vi "CRYSet Import Calibration Data Dialog Front Panel.vi"(11 "Vi Ref":refnum<vi>) -> ()   [LabVIEW 2013]
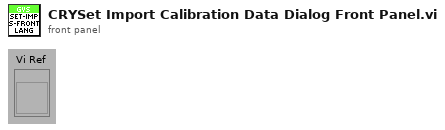
[diagram p1: front panel]
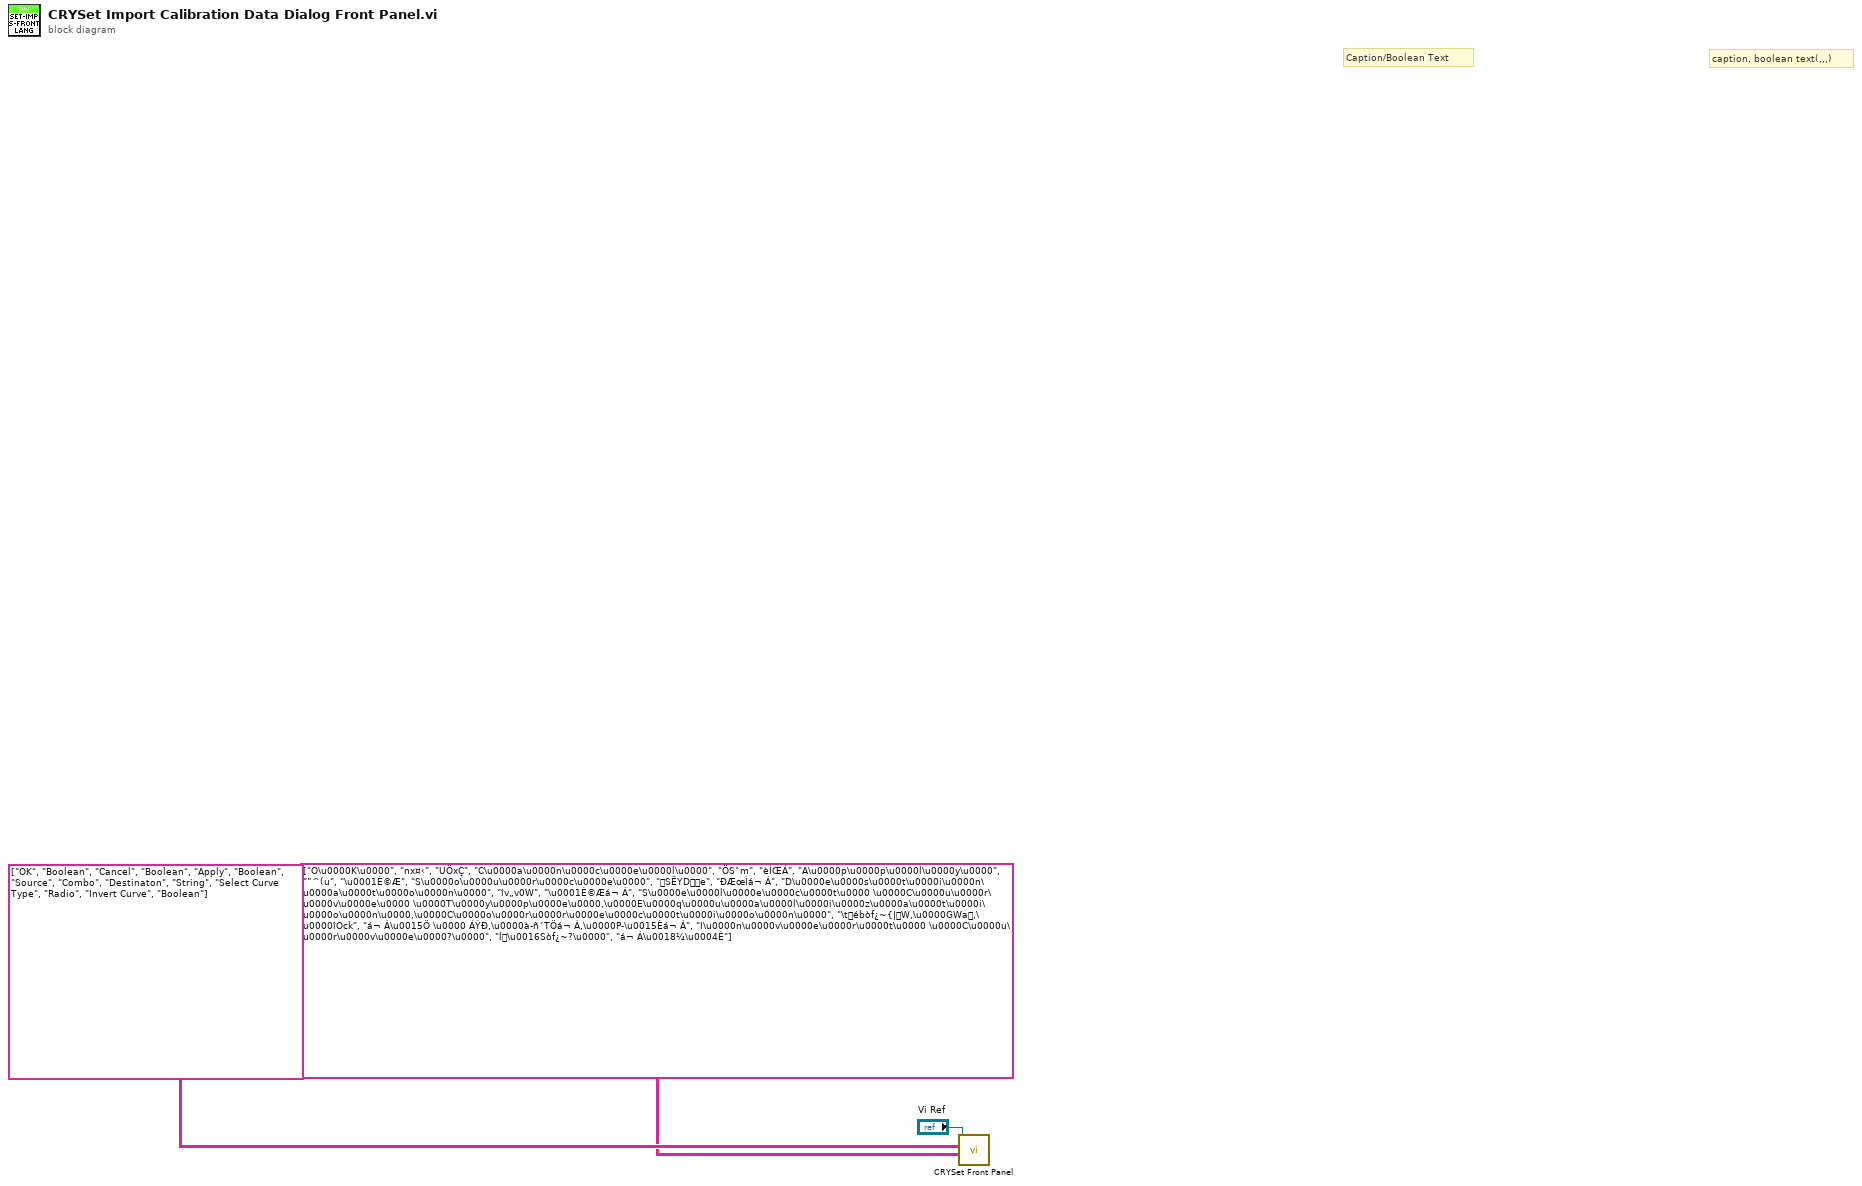
[diagram p0: block diagram]
diagram:
  # "caption, boolean text(,,,)"
  # "Caption/Boolean Text"
  n1 = call "CRYSet Front Panel.vi"("Caption(Boolean Text)"=string[][] [["O\u0000K\u0000", "nx¤‹", "UÖxÇ"], ["C\u0000a\u0000n\u0000c\u0000e\u0000l\u0000", "ÖSˆm", "èÍŒÁ"], ["A\u0000p\u0000p\u0000l\u0000y\u0000", "”^(u", "\u0001È©Æ"], ["S\u0000o\u0000u\u0000r\u0000c\u0000e\u0000", "SËYDe", "ÐÆœÌá¬ Á"], ["D\u0000e\u0000s\u0000t\u0000i\u0000n\u0000a\u0000t\u0000o\u0000n\u0000", "îv„v0W", "\u0001È©Æá¬ Á"], ["S\u0000e\u0000l\u0000e\u0000c\u0000t\u0000 \u0000C\u0000u\u0000r\u0000v\u0000e\u0000 \u0000T\u0000y\u0000p\u0000e\u0000,\u0000E\u0000q\u0000u\u0000a\u0000l\u0000i\u0000z\u0000a\u0000t\u0000i\u0000o\u0000n\u0000,\u0000C\u0000o\u0000r\u0000r\u0000e\u0000c\u0000t\u0000i\u0000o\u0000n\u0000", "\tébòf¿~{|W,\u0000GWa,\u0000îOck", "á¬ Á\u0015Ö \u0000 ÁÝÐ,\u0000à­ñ´TÖá¬ Á,\u0000P­\u0015Èá¬ Á"], ["I\u0000n\u0000v\u0000e\u0000r\u0000t\u0000 \u0000C\u0000u\u0000r\u0000v\u0000e\u0000?\u0000", "l\u0016Sòf¿~?\u0000", "á¬ Á\u0018¼\u0004È"]], "Control ID and Type(Label Name, Type)"=string[][] [["OK", "Boolean"], ["Cancel", "Boolean"], ["Apply", "Boolean"], ["Source", "Combo"], ["Destinaton", "String"], ["Select Curve Type", "Radio"], ["Invert Curve", "Boolean"]], "Vi Ref"="Vi Ref") -> ()  [unwired: 9 in]
